vi "InTake Get.vi"(1 "UpperClaw":dbl, 2 "TakeBall":dbl) -> ()   [LabVIEW 2013]
uses:
  InTake Global Data.vi
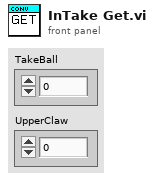
[diagram p1: front panel]
types:
  T1 = cluster{"TakeBall":dbl, "UpperClaw":dbl, "MS":bool, "Upper claw max":bool, "Upper claw min":bool, "Angle":dbl}
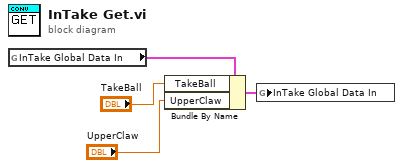
[diagram p0: block diagram]
diagram:
  n1 = global read "InTake Global Data.vi" "InTake Global Data In"() -> (w4:T1)
  n2 = Bundle By Name(cluster=w4, "TakeBall"="TakeBall", "UpperClaw"="UpperClaw") -> (w3:T1)
  n3 = global write "InTake Global Data.vi" "InTake Global Data In"(w3) -> ()
